vi "DecisionMaker.vi"(8 "Goal location":T3 {"North" format="%#_10f"; "East" format="%#_8f"}, 9 "Heading to test":dbl) -> (1 "Heading Goodness":T1)   [LabVIEW 2011]
doc: "VI to make decisions when the boat is headed upwind.\n\nCalculates the vector that goes to the goal from the boat's current location when first called.\nConstantly calculates the two optimal angles with respect to the wind and gives one of them as the optimal angle. On first call, this will be the one that is closer to the robot's current heading. It also calculates the distance from the boat to the original line calculated. If the distance gets larger than the allowed distance, it switches the angle outputted as optimal to the other angle that is good with respect to the wind."
uses:
  2 Typedefs/apparent wind direction.ctl
  2 Globals/2 Global.vi
  2 Globals/2 TuningConstants.vi
panel:
  in  "Aggressiveness":dbl min=0.0 max=1.0
  in  "Irons direct vector":T2 {"Origin"."North" format="%#_10f"; "Origin"."East" format="%#_8f"}
  in  "Already Upwind?":bool
  # "0 < A < 1"
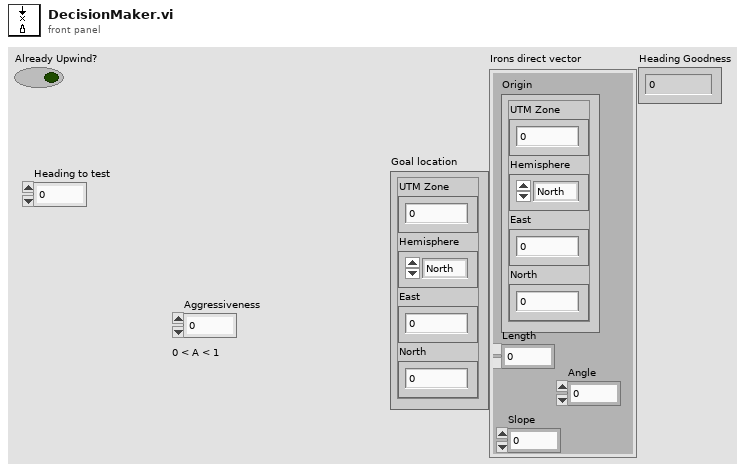
[diagram p1: front panel]
types:
  T1 = typedef "apparent wind direction.ctl" = dbl
  T2 = cluster{"Origin":cluster{"UTM Zone":dbl, "Hemisphere":enum16{"North", "South"}, "East":dbl, "North":dbl}, "Length":dbl, "Angle":dbl, "Slope":dbl}
  T3 = cluster{"UTM Zone":dbl, "Hemisphere":enum16{"North", "South"}, "East":dbl, "North":dbl}
  T4 = typedef "UTM Location.ctl" = cluster{"UTM Zone":dbl, "Hemisphere":enum16{"North", "South"}, "East":dbl, "North":dbl}
  T5 = cluster{"UTM Zone":bool, "Hemisphere":bool, "East":bool, "North":bool}
  T6 = typedef "heading.ctl" = dbl
  T7 = typedef "absolute wind direction.ctl" = dbl
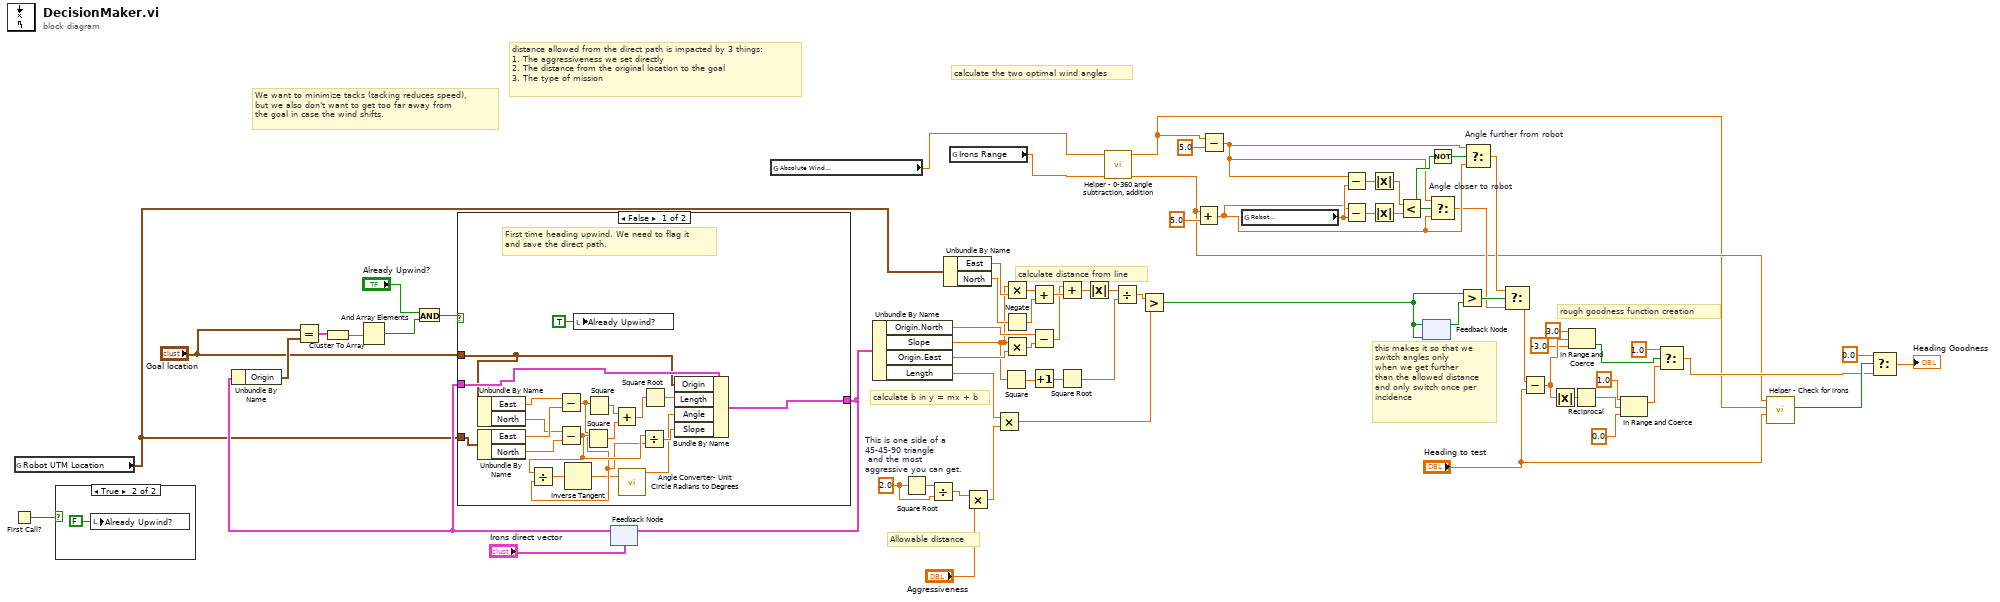
[diagram p0: block diagram]
diagram:
  w39 = 2.0 ("x")
  # "Allowable distance"
  # "rough goodness function creation"
  # "this makes it so that we\nswitch angles only\nwhen we get further\nthan the allowed distance\nand only switch once per\nincidence"
  # "calculate distance from line"
  # "calculate the two optimal wind angles"
  # "calculate b in y = mx + b"
  # "distance allowed from the direct path is impacted by 3 things:\n1. The aggressiveness we set directly\n2. The distance from the original location to the goal\n3. The type of mission"
  # "We want to minimize tacks (tacking reduces speed),\nbut we also don't want to get too far away from\nthe goal in case the wind shifts."
  n1 = First Call?() -> (First Call?: T/F=w38:bool)
  n2 = global read "2 Global.vi" "Robot UTM Location"() -> (w23:T4)
  n3 = case shown="True" w38 {
    frame False {
    }
    frame True {
      n4 = local write "Already Upwind?"(FALSE ("Already Upwind?")) -> ()
    }
  }
  n5 = feedback #1("Irons direct vector") -> (w35:T2)
  n6 = Unbundle By Name(w35) -> ("Origin"=w34:T3)
  n7 = Equal?(x="Goal location", y=w34) -> (x = y?=w33:T5)
  n8 = Cluster To Array(cluster=w33) -> (array=w32:bool[])
  n9 = And Array Elements(Boolean array=w32) -> (logical AND=w31:bool)
  n10 = And(x="Already Upwind?", y=w31) -> (x .and. y?=w37:bool)
  n11 = case shown="False" w37 {
    tunnel: w35 -> [w90 w92]
    tunnel: "Goal location" -> [w85 _]
    tunnel: w23 -> [w84 _]
    tunnel: [w78 w92] -> w55
    frame False {
      # "First time heading upwind. We need to flag it\nand save the direct path."
      n12 = Unbundle By Name(w85) -> ("East"=w83:dbl, "North"=w81:dbl)
      n13 = Unbundle By Name(w84) -> ("East"=w82:dbl, "North"=w80:dbl)
      n14 = Subtract(x=w83, y=w82) -> (x-y=w75:dbl)
      n15 = Subtract(x=w81, y=w80) -> (x-y=w76:dbl)
      n16 = Divide(x=w76, y=w75) -> (x/y=w79:dbl)
      n17 = Inverse Tangent(1:w79) -> (0:w74:dbl)
      n18 = local write "Already Upwind?"(TRUE ("Already Upwind?")) -> ()
      n19 = Square(x=w76) -> (x^2=w88:dbl)
      n20 = Square(x=w75) -> (x^2=w89:dbl)
      n21 = Add(x=w89, y=w88) -> (x+y=w86:dbl)
      n22 = call "Angle Converter- Unit Circle Radians to Degrees.vi"("Angle in \nUnit Circle\nRadians"=w74) -> ("Angle in \nHeading \nFormat"=w73:T6)  [unwired: 10 in]
      n23 = Divide(x=w76, y=w75) -> (x/y=w77:dbl)
      n24 = Square Root(x=w86) -> (sqrt(x)=w87:dbl)
      n25 = Bundle By Name(cluster=w90, "Origin"=w85, "Length"=w87, "Angle"=w73, "Slope"=w77) -> (w78:T2)
    }
    frame True {
    }
  }
  n26 = feedback-in #1(w55) -> ()
  n27 = global read "2 Global.vi" "Absolute Wind\nDirection (º)"() -> (w6:T7)
  n28 = Unbundle By Name(w55) -> ("Origin.North"=w70:dbl, "Slope"=w58:dbl, "Origin.East"=w69:dbl, "Length"=w42:dbl)
  n29 = Square Root(x=w39) -> (sqrt(x)=w40:dbl)
  n30 = Divide "This is one side of a 45-45-90 triangle\n and the most aggressive you can get."(x=w40, y=w39) -> (x/y=w3:dbl)
  n31 = Unbundle By Name(w23) -> ("East"=w67:dbl, "North"=w65:dbl)
  n32 = global read "2 TuningConstants.vi" "Irons Range"() -> (w7:dbl)
  n33 = Multiply(x=w3, y="Aggressiveness") -> (x*y=w1:dbl)
  n34 = Multiply(x=w42, y=w1) -> (x*y=w41:dbl)
  n35 = Square(x=w58) -> (x^2=w57:dbl)
  n36 = Multiply(x=w58, y=w67) -> (x*y=w66:dbl)
  n37 = Negate(x=w65) -> (-x=w64:dbl)
  n38 = Multiply(x=w58, y=w69) -> (x*y=w68:dbl)
  n39 = Add(x=w66, y=w64) -> (x+y=w63:dbl)
  n40 = Subtract(x=w70, y=w68) -> (x-y=w62:dbl)
  n41 = Increment(x=w57) -> (x+1=w56:dbl)
  n42 = Add(x=w62, y=w63) -> (x+y=w61:dbl)
  n43 = Square Root(x=w56) -> (sqrt(x)=w59:dbl)
  n44 = Absolute Value(x=w61) -> (abs(x)=w60:dbl)
  n45 = call "Helper - 0-360 angle subtraction, addition.vi"("y"=w7, "x"=w6) -> ("x + y"=w5:dbl, "x - y"=w4:T1)  [unwired: 8 in]
  n46 = Divide(x=w60, y=w59) -> (x/y=w54:dbl)
  n47 = Greater?(x=w54, y=w41) -> (0:w16:bool)
  n48 = Add(x=w5, y=T1 5.0) -> (x+y=w10:T1)
  n49 = Subtract(x=w4, y=T1 5.0) -> (x-y=w11:T1)
  n50 = global read "2 Global.vi" "Robot\nHeading"() -> (w21:T6)
  n51 = Subtract(x=w11, y=w21) -> (x-y=w20:T1)
  n52 = Subtract(x=w10, y=w21) -> (x-y=w19:T1)
  n53 = Absolute Value(x=w20) -> (abs(x)=w18:T1)
  n54 = Absolute Value(x=w19) -> (abs(x)=w17:T1)
  n55 = Less?(x=w18, y=w17) -> (x < y?=w12:bool)
  n56 = feedback-in #2(w16) -> ()
  n57 = feedback #2(w16) -> (w15:bool)
  n58 = Not(x=w12) -> (.not. x?=w13:bool)
  n59 = Select "Angle closer to robot"(t=w11, s=w12, f=w10) -> (s? t:f=w8:T1)
  n60 = Greater?(x=w16, y=w15) -> (0:w14:bool)
  n61 = Select "Angle further from robot"(t=w11, s=w13, f=w10) -> (s? t:f=w9:T1)
  n62 = Select(t=w9, s=w14, f=w8) -> (s? t:f=w53:T1)
  n63 = Subtract(x=w53, y="Heading to test") -> (x-y=w28:T1)
  n64 = Absolute Value(x=w28) -> (abs(x)=w51:T1)
  n65 = In Range and Coerce(upper limit=T1 3.0, x=w28, lower limit=T1 -3.0) -> (In Range?=w25:bool)  [unwired: 1 out]
  n66 = Reciprocal(x=w51) -> (1/x=w49:T1)
  n67 = In Range and Coerce(upper limit=T1 1.0, x=w49, lower limit=T1 0.0) -> (coerced(x)=w30:T1)  [unwired: 1 out]
  n68 = Select(t=1.0, s=w25, f=w30) -> (s? t:f=w29:T1)
  n69 = call "Helper - Check for irons.vi"("Angle to check"="Heading to test", "Wind - Irons range"=w4, "Wind + Irons range"=w5) -> ("In irons?"=w46:bool)  [unwired: 8 in]
  n70 = Select(t=0.0, s=w46, f=w29) -> (s? t:f=→"Heading Goodness":T1)
